vi "Initalize SR830(SubVI).vi"(0 "队列输入":refnum<queue>, 9 "字符串":string) -> ()   [LabVIEW 2019, in "SubVI.lvlib"]
uses:
  SubVI.lvlib
  lib/Keithley 622x/Configure/6221 Wave/Typedefs/KE6221 -- Wave Sine Wave Params.ctl
  lib/Keithley 622x/Configure/6221 Wave/Low Level/Typedefs/KE6221 -- Wave Frequency.ctl
  lib/Keithley 622x/Configure/6221 Wave/Low Level/Typedefs/KE6221 -- Wave Amplitude.ctl
  lib/Keithley 622x/Configure/Source/Typedefs/KE622x -- Current Level.ctl
  lib/Keithley 622x/Configure/6221 Wave/Low Level/Typedefs/KE6221 -- Wave Ranging Mode.ctl
  lib/Keithley 622x/Configure/Source/Typedefs/KE622x -- Current Ranges.ctl
  lib/Keithley 622x/Configure/6221 Wave/Low Level/Typedefs/KE6221 -- Wave Playback Mode.ctl
  lib/Keithley 622x/Configure/6221 Wave/Low Level/Typedefs/KE6221 -- Wave Playback Time.ctl
  lib/Keithley 622x/Configure/6221 Wave/Low Level/Typedefs/KE6221 -- Wave Playback Num Cycles.ctl
  lib/Keithley 622x/Configure/6221 Wave/Low Level/Typedefs/KE6221 -- Wave Phase Marker.ctl
  lib/Keithley 622x/Configure/Trigger/Low Level/Typedefs/KE622x -- Trig Link Line.ctl
  error.ctl
  lib/QDInstrument.dll
  lib/Keithley 622x/Configure/6221 Wave/Low Level/Typedefs/KE6221 -- Wave Type.ctl
  lib/Keithley 622x/Keithley 622x.lvlib
panel:
  out "x/y":dbl
  in  "6221(SR830做源可忽略）":T12={"Sine Wave Params In"={"Frequency (Hz)"=1000.0, "Amplitude (A)"=0.001, "Offset (A)"=0.0, "Ranging Mode"=enum."Best", "Fixed Range"=enum."2mA", "Playback Mode"=enum."Time", "Time (s)"=999999.999, "Num Cycles"=1.0, "Phase\nMarker?"=FALSE, "Phase Marker (deg)"=180.0, "Trig Link Line"=enum."1"}, "RMS Amplitude (A)"=0.001, "6221 resource"=""} {"RMS Amplitude (A)" min=2e-12 max=0.105 format="%.3p"; "Sine Wave Params In"."Offset (A)" min=-0.105 max=0.105 format="%.4p"; "Sine Wave Params In"."Num Cycles" min=0.001 max=99999999900.0 format="%.3p"; "Sine Wave Params In"."Time (s)" min=1e-07 max=999999.999 format="%.3p"; "Sine Wave Params In"."Phase Marker (deg)" min=0.0 max=360.0 format="%.3f"; "Sine Wave Params In"."Amplitude (A)" min=2e-12 max=0.105 format="%.3p"; "Sine Wave Params In"."Frequency (Hz)" min=0.001 max=100000.0 format="%.3p"}
  in  "仪器设置":T13={"ID Query"=FALSE, "Reset"=FALSE, "VISA 1"="", "VISA 2"="", "VISA 3"="", "VISA 4"="", "Sensitivity 2"=-1, "Sensitivity 1"=-1, "量程"=enum."量程每次测量会判定", "SR830源配合的阻抗（6221做源可忽略）"=0.0, "SR830 2"=FALSE, "SR830 3"=FALSE, "SR830 4"=FALSE, "Sensitivity 3"=-1, "Sensitivity 4"=-1, "source"=0, "SR830 1"=FALSE} {"source" items=["SR830 1", "SR830 2", "SR830 3", "SR830 4"]; "Sensitivity 4" items=["Auto Gain"=-1, "2 nV/fA"=0, "5 nV/fA"=1, "10 nV/fA"=2, "20 nV/fA"=3, "50 nV/fA"=4, "100 nV/fA"=5, "200 nV/fA"=6, "500 nV/fA"=7, "1 uV/pA"=8, "2 uV/pA"=9, "5 uV/pA"=10, "10 uV/pA"=11, "20 uV/pA"=12, "50 uV/pA"=13, "100 uV/pA"=14, "200 uV/pA"=15, "500 uV/pA"=16, "1 mV/nA"=17, "2 mV/nA"=18, "5 mV/nA"=19, "10 mV/nA"=20, "20 mV/nA"=21, "50 mV/nA"=22, "100 mV/nA"=23, "200 mV/nA"=24, "500 mV/mA"=25, "1 V/uA"=26]; "Sensitivity 3" items=["Auto Gain"=-1, "2 nV/fA"=0, "5 nV/fA"=1, "10 nV/fA"=2, "20 nV/fA"=3, "50 nV/fA"=4, "100 nV/fA"=5, "200 nV/fA"=6, "500 nV/fA"=7, "1 uV/pA"=8, "2 uV/pA"=9, "5 uV/pA"=10, "10 uV/pA"=11, "20 uV/pA"=12, "50 uV/pA"=13, "100 uV/pA"=14, "200 uV/pA"=15, "500 uV/pA"=16, "1 mV/nA"=17, "2 mV/nA"=18, "5 mV/nA"=19, "10 mV/nA"=20, "20 mV/nA"=21, "50 mV/nA"=22, "100 mV/nA"=23, "200 mV/nA"=24, "500 mV/mA"=25, "1 V/uA"=26]; "Sensitivity 1" items=["Auto Gain"=-1, "2 nV/fA"=0, "5 nV/fA"=1, "10 nV/fA"=2, "20 nV/fA"=3, "50 nV/fA"=4, "100 nV/fA"=5, "200 nV/fA"=6, "500 nV/fA"=7, "1 uV/pA"=8, "2 uV/pA"=9, "5 uV/pA"=10, "10 uV/pA"=11, "20 uV/pA"=12, "50 uV/pA"=13, "100 uV/pA"=14, "200 uV/pA"=15, "500 uV/pA"=16, "1 mV/nA"=17, "2 mV/nA"=18, "5 mV/nA"=19, "10 mV/nA"=20, "20 mV/nA"=21, "50 mV/nA"=22, "100 mV/nA"=23, "200 mV/nA"=24, "500 mV/mA"=25, "1 V/uA"=26]; "Sensitivity 2" items=["Auto Gain"=-1, "2 nV/fA"=0, "5 nV/fA"=1, "10 nV/fA"=2, "20 nV/fA"=3, "50 nV/fA"=4, "100 nV/fA"=5, "200 nV/fA"=6, "500 nV/fA"=7, "1 uV/pA"=8, "2 uV/pA"=9, "5 uV/pA"=10, "10 uV/pA"=11, "20 uV/pA"=12, "50 uV/pA"=13, "100 uV/pA"=14, "200 uV/pA"=15, "500 uV/pA"=16, "1 mV/nA"=17, "2 mV/nA"=18, "5 mV/nA"=19, "10 mV/nA"=20, "20 mV/nA"=21, "50 mV/nA"=22, "100 mV/nA"=23, "200 mV/nA"=24, "500 mV/mA"=25, "1 V/uA"=26]}
  out "错误输出":errorcluster
  in  "滤波设置 4":T14={"Time Constant "=8, "Low Pass Filter Slope "=1, "Enable Sync Filter "=TRUE} {"Low Pass Filter Slope" items=["6 dB/oct", "12 dB/oct", "18 db/oct", "24 dB/oct"]; "Time Constant" items=["10 us", "30 us", "100 us", "300 us", "1 ms", "3 ms", "10 ms", "30 ms", "100 ms", "300 ms", "1 s", "3 s", "10 s", "30 s", "100 s", "300 s", "1 ks", "3 ks", "10 ks", "30 ks"]}
  in  "滤波设置 3":T14={"Time Constant "=8, "Low Pass Filter Slope "=1, "Enable Sync Filter "=TRUE} {"Low Pass Filter Slope" items=["6 dB/oct", "12 dB/oct", "18 db/oct", "24 dB/oct"]; "Time Constant" items=["10 us", "30 us", "100 us", "300 us", "1 ms", "3 ms", "10 ms", "30 ms", "100 ms", "300 ms", "1 s", "3 s", "10 s", "30 s", "100 s", "300 s", "1 ks", "3 ks", "10 ks", "30 ks"]}
  in  "滤波设置 2":T14={"Time Constant "=8, "Low Pass Filter Slope "=1, "Enable Sync Filter "=TRUE} {"Low Pass Filter Slope" items=["6 dB/oct", "12 dB/oct", "18 db/oct", "24 dB/oct"]; "Time Constant" items=["10 us", "30 us", "100 us", "300 us", "1 ms", "3 ms", "10 ms", "30 ms", "100 ms", "300 ms", "1 s", "3 s", "10 s", "30 s", "100 s", "300 s", "1 ks", "3 ks", "10 ks", "30 ks"]}
  in  "参考信号 4":T15={"Reference Source"=1, "External Reference Trigger  "=0, "Detection Harmonic Number "=1.0, "Manual Phase (Degree)"=0.0, "Auto Phase "=FALSE, "Sine Output Amplitude (V)"=1.0, "Internal Reference Frequency (Hz)"=13.0} {"External Reference Trigger" items=["Sine Zero Crossing", "TTL Rising Edge", "TTL Falling Edge"]; "Reference Source" items=["External", "Internal"]}
  in  "参考信号 3":T15={"Reference Source"=1, "External Reference Trigger  "=0, "Detection Harmonic Number "=1.0, "Manual Phase (Degree)"=0.0, "Auto Phase "=FALSE, "Sine Output Amplitude (V)"=1.0, "Internal Reference Frequency (Hz)"=13.0} {"External Reference Trigger" items=["Sine Zero Crossing", "TTL Rising Edge", "TTL Falling Edge"]; "Reference Source" items=["External", "Internal"]}
  in  "参考信号 2":T15={"Reference Source"=1, "External Reference Trigger  "=0, "Detection Harmonic Number "=1.0, "Manual Phase (Degree)"=0.0, "Auto Phase "=FALSE, "Sine Output Amplitude (V)"=1.0, "Internal Reference Frequency (Hz)"=13.0} {"External Reference Trigger" items=["Sine Zero Crossing", "TTL Rising Edge", "TTL Falling Edge"]; "Reference Source" items=["External", "Internal"]}
  in  "输入信号 4":T16={"Input Notch Filter "=0, "Input Shield Grounding"=0, "Input Coupling "=0, "Input Connection  "=1} {"Input Connection" items=["Single-Ended Voltage", "Differential Voltage", "1 MOhm Current Gain", "100 MOhm Current Gain"]; "Input Coupling" items=["AC", "DC"]; "Input Shield Grounding" items=["Float", "Ground"]; "Input Notch Filter" items=["None", "Line Notch", "2x Line Notch", "Both Notch Filters"]}
  in  "输入信号 3":T16={"Input Notch Filter "=0, "Input Shield Grounding"=0, "Input Coupling "=0, "Input Connection  "=1} {"Input Connection" items=["Single-Ended Voltage", "Differential Voltage", "1 MOhm Current Gain", "100 MOhm Current Gain"]; "Input Coupling" items=["AC", "DC"]; "Input Shield Grounding" items=["Float", "Ground"]; "Input Notch Filter" items=["None", "Line Notch", "2x Line Notch", "Both Notch Filters"]}
  in  "输入信号 2":T16={"Input Notch Filter "=0, "Input Shield Grounding"=0, "Input Coupling "=0, "Input Connection  "=1} {"Input Connection" items=["Single-Ended Voltage", "Differential Voltage", "1 MOhm Current Gain", "100 MOhm Current Gain"]; "Input Coupling" items=["AC", "DC"]; "Input Shield Grounding" items=["Float", "Ground"]; "Input Notch Filter" items=["None", "Line Notch", "2x Line Notch", "Both Notch Filters"]}
  in  "滤波设置":T14={"Time Constant "=8, "Low Pass Filter Slope "=1, "Enable Sync Filter "=TRUE} {"Low Pass Filter Slope" items=["6 dB/oct", "12 dB/oct", "18 db/oct", "24 dB/oct"]; "Time Constant" items=["10 us", "30 us", "100 us", "300 us", "1 ms", "3 ms", "10 ms", "30 ms", "100 ms", "300 ms", "1 s", "3 s", "10 s", "30 s", "100 s", "300 s", "1 ks", "3 ks", "10 ks", "30 ks"]}
  in  "参考信号":T15={"Reference Source"=1, "External Reference Trigger  "=0, "Detection Harmonic Number "=1.0, "Manual Phase (Degree)"=0.0, "Auto Phase "=FALSE, "Sine Output Amplitude (V)"=1.0, "Internal Reference Frequency (Hz)"=13.0} {"External Reference Trigger" items=["Sine Zero Crossing", "TTL Rising Edge", "TTL Falling Edge"]; "Reference Source" items=["External", "Internal"]}
  in  "输入信号":T16={"Input Notch Filter "=0, "Input Shield Grounding"=0, "Input Coupling "=0, "Input Connection  "=1} {"Input Connection" items=["Single-Ended Voltage", "Differential Voltage", "1 MOhm Current Gain", "100 MOhm Current Gain"]; "Input Coupling" items=["AC", "DC"]; "Input Shield Grounding" items=["Float", "Ground"]; "Input Notch Filter" items=["None", "Line Notch", "2x Line Notch", "Both Notch Filters"]}
  # "(真是通道1，假是通道2)"
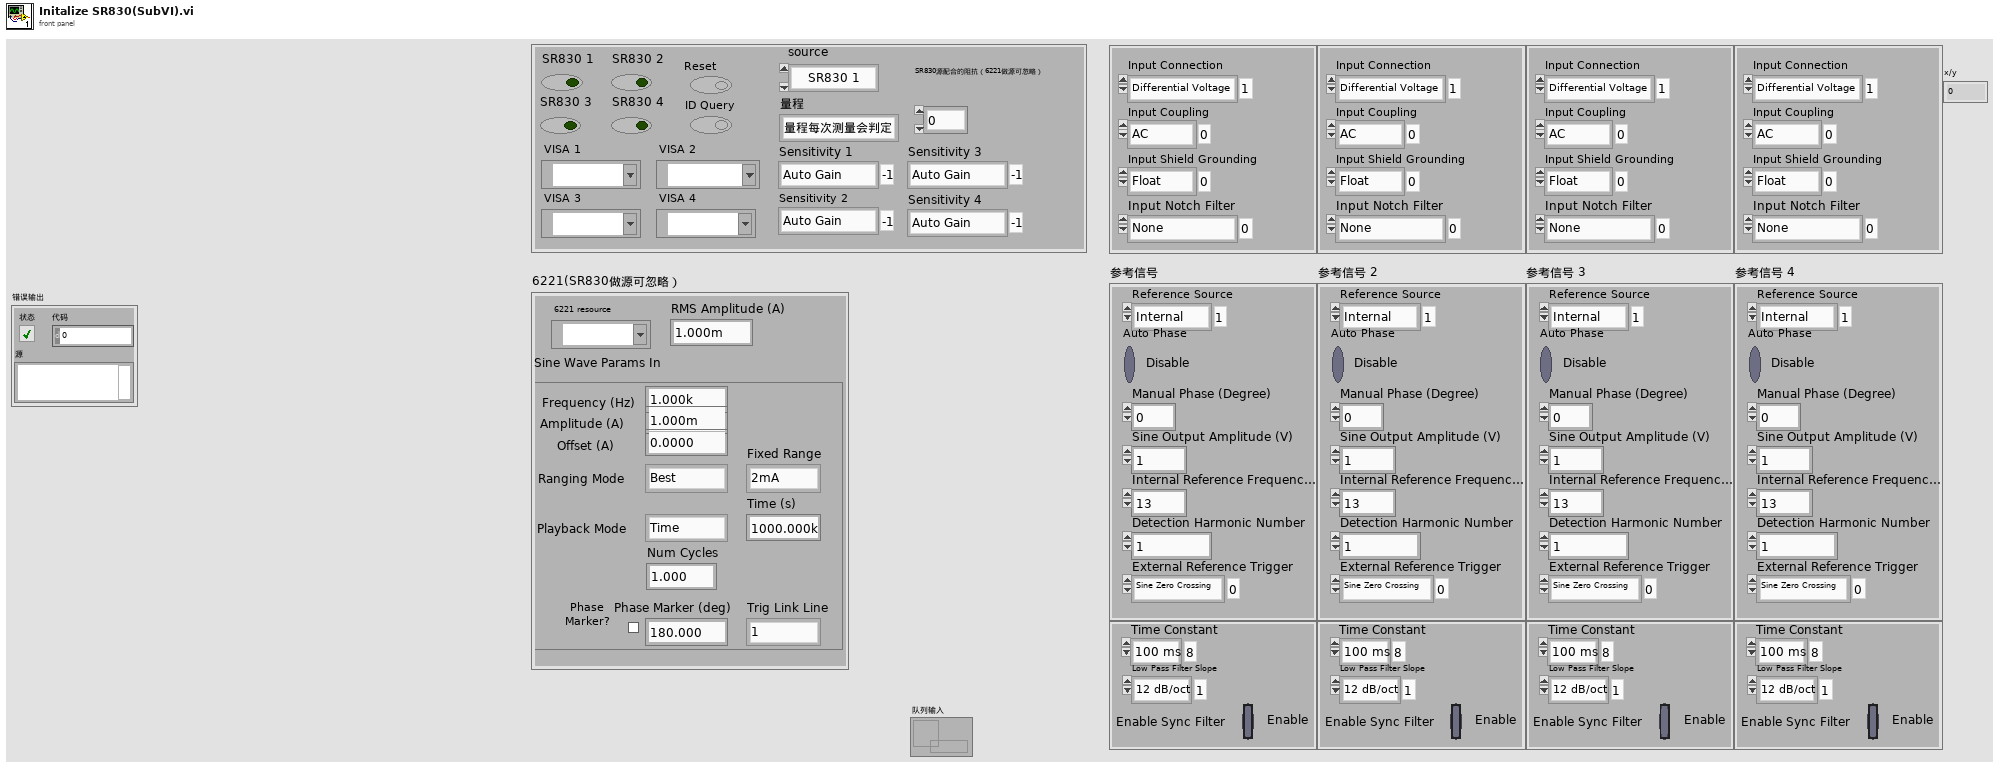
[diagram p1: front panel]
types:
  T1 = typedef "Keithley 622x.lvlib/KE6221 -- Wave Sine Wave Params.ctl" = cluster{"Frequency (Hz)":T2, "Amplitude (A)":T3, "Offset (A)":T4, "Ranging Mode":T5, "Fixed Range":T6, "Playback Mode":T7, "Time (s)":T8, "Num Cycles":T9, "Phase\nMarker?":bool, "Phase Marker (deg)":T10, "Trig Link Line":T11}
  T2 = typedef "Keithley 622x.lvlib/KE6221 -- Wave Frequency.ctl" = dbl
  T3 = typedef "Keithley 622x.lvlib/KE6221 -- Wave Amplitude.ctl" = dbl
  T4 = typedef "Keithley 622x.lvlib/KE622x -- Current Level.ctl" = dbl
  T5 = typedef "Keithley 622x.lvlib/KE6221 -- Wave Ranging Mode.ctl" = enum16{"Best", "Fixed"}
  T6 = typedef "Keithley 622x.lvlib/KE622x -- Current Ranges.ctl" = enum16{"2nA", "20nA", "200nA", "2uA", "20uA", "200uA", "2mA", "20mA", "100mA"}
  T7 = typedef "Keithley 622x.lvlib/KE6221 -- Wave Playback Mode.ctl" = enum16{"Time", "Num Cycles"}
  T8 = typedef "Keithley 622x.lvlib/KE6221 -- Wave Playback Time.ctl" = dbl
  T9 = typedef "Keithley 622x.lvlib/KE6221 -- Wave Playback Num Cycles.ctl" = dbl
  T10 = typedef "Keithley 622x.lvlib/KE6221 -- Wave Phase Marker.ctl" = dbl
  T11 = typedef "Keithley 622x.lvlib/KE622x -- Trig Link Line.ctl" = enum16{"1", "2", "3", "4", "5", "6"}
  T12 = cluster{"Sine Wave Params In":T1, "RMS Amplitude (A)":T3, "6221 resource":refnum<visa-resource-name>}
  T13 = cluster{"ID Query":bool, "Reset":bool, "VISA 1":refnum<visa-resource-name>, "VISA 2":refnum<visa-resource-name>, "VISA 3":refnum<visa-resource-name>, "VISA 4":refnum<visa-resource-name>, "Sensitivity 2":i16, "Sensitivity 1":i16, "量程":enum16{"量程每次测量会判定", "量程不变为设定值"}, "SR830源配合的阻抗（6221做源可忽略）":dbl, "SR830 2":bool, "SR830 3":bool, "SR830 4":bool, "Sensitivity 3":i16, "Sensitivity 4":i16, "source":u16, "SR830 1":bool}
  T14 = cluster{"Time Constant ":u16, "Low Pass Filter Slope ":u16, "Enable Sync Filter ":bool}
  T15 = cluster{"Reference Source":u16, "External Reference Trigger  ":u16, "Detection Harmonic Number ":dbl, "Manual Phase (Degree)":dbl, "Auto Phase ":bool, "Sine Output Amplitude (V)":dbl, "Internal Reference Frequency (Hz)":dbl}
  T16 = cluster{"Input Notch Filter ":u16, "Input Shield Grounding":u16, "Input Coupling ":u16, "Input Connection  ":u16}
  T17 = enum16{"open", "replace", "create", "open or create", "replace or create", "replace or create with confirmation"}
  T18 = typedef "Keithley 622x.lvlib/KE6221 -- Wave Type.ctl" = enum16{"Sinusoid", "Square", "Ramp", "Arbitrary 0", "Arbitrary 1", "Arbitrary 2", "Arbitrary 3", "Arbitrary 4"}
  T19 = typedef "Keithley 622x.lvlib/KE622x -- On Off Control.ctl" = enum16{"Off", "On"}
  T20 = typedef "error.ctl" = cluster{"initialize":string, "6221":cluster{"6221 Resource":refnum<visa-resource-name>, "Delta status":bool}, "7001":cluster{"Ch":bool}, "SR830+6221":cluster{"source":u16, "阻抗":dbl, "量程入 4":i32, "量程入 3":i32, "量程入 2":i32, "量程入 1":i32, "电流":dbl, "SR830 2":bool, "SR830 3":bool, "SR830 4":bool, "SR830 1":bool, "VISA 1":refnum<visa-resource-name>, "VISA 2":refnum<visa-resource-name>, "VISA 3":refnum<visa-resource-name>, "VISA 4":refnum<visa-resource-name>, "量程":enum16{"量程每次测量会判定", "量程不变为设定值"}}, "2400":cluster{"2400":bool, "VISA":refnum<visa-resource-name>}, "ch":cluster{"ch str":string, "ch1":bool, "ch2":bool, "布尔":bool}, "quantum design":refnum<k24>, "error":bool, "数据文件路径":path, "簇":cluster{"log路径":path, "log interval":dbl}}
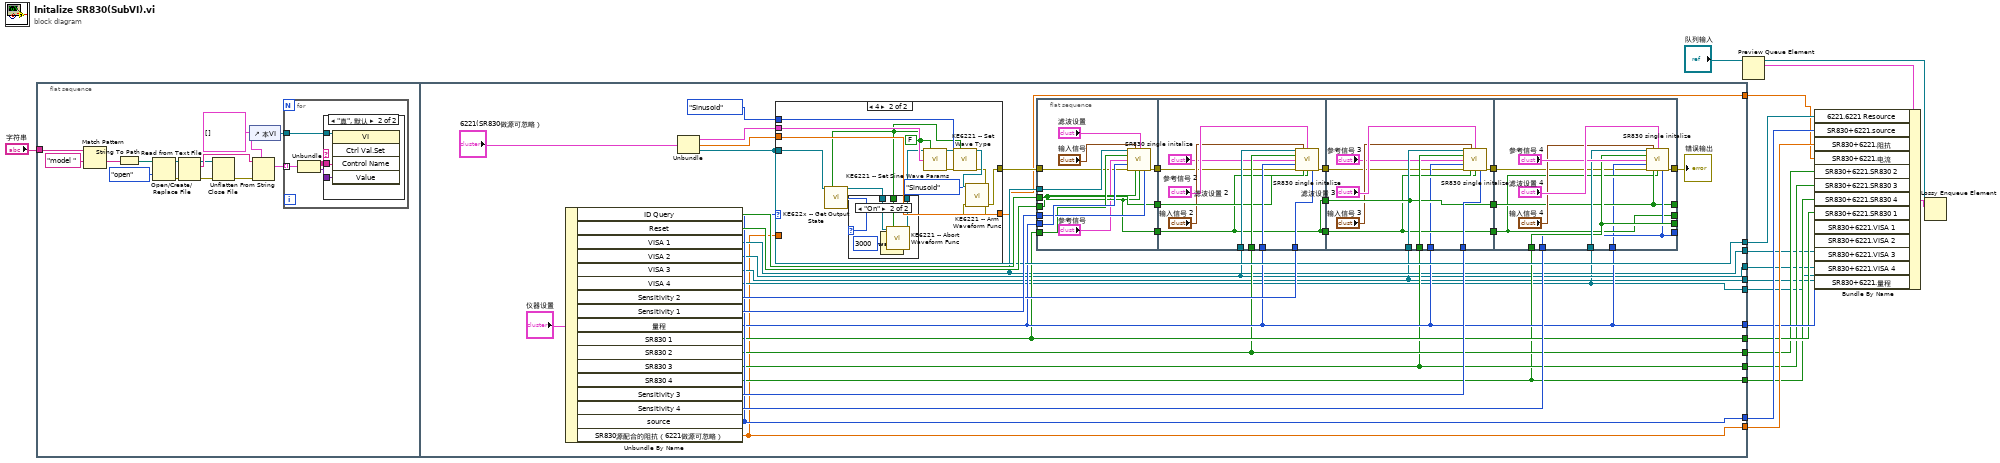
[diagram p0: block diagram]
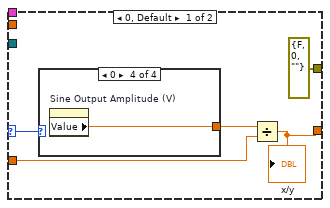
[diagram p3: hidden frame]
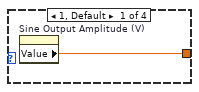
[diagram p4: hidden frame]
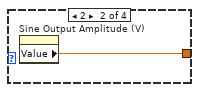
[diagram p5: hidden frame]
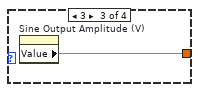
[diagram p6: hidden frame]
diagram:
  n1 = flat-sequence {
    tunnel: "字符串" -> [w32]
    tunnel: [w56] -> w13
    tunnel: [w53] -> w14
    tunnel: [w41] -> w12
    tunnel: [w51] -> w10
    tunnel: [w50] -> w9
    tunnel: [w49] -> w8
    tunnel: [w48] -> w7
    tunnel: [w47] -> w6
    tunnel: [w46] -> w5
    tunnel: [w45] -> w4
    tunnel: [w44] -> w3
    tunnel: [w43] -> w2
    tunnel: [w40] -> w1
    frame #0 {
      n2 = Match Pattern(string=w32, regular expression="model " ("正则表达式")) -> (after substring=w31:string)  [unwired: 1 in, 3 out]
      n3 = String To Path(string=w31) -> (path=w30:path)
      n4 = Open/Create/Replace File(file path (use dialog)=w30, operation (0:open)=T17."open" ("操作(0:open)")) -> (refnum out=w27:refnum<file>, error out=w25:errorcluster)  [unwired: 4 in, 1 out]
      n5 = Read from Text File(file (use dialog)=w27, error in=w25) -> (refnum out=w26:refnum<file>, text=w28:string, error out=w24:errorcluster)  [unwired: 2 in, 1 out]
      n6 = Close File(refnum=w26, error in=w24) -> (error out=w23:errorcluster)  [unwired: 1 out]
      n7 = control-ref of="本VI"() -> (w19:refnum<vi>)
      n8 = Unflatten From String(type=cluster{"Name":string, "Variant Data":variant}[] [] ("控件值:获取全部"), binary string=w28, error in (no error)=w23) -> (value=w20:cluster{"Name":string, "Variant Data":variant}[])  [unwired: 2 in, 2 out]
      n9 = for {
        tunnel: w20 -> [w36] mode=indexing
        tunnel: w19 -> [w35]
        n10 = Unbundle(w36) -> ("Name"=w33:string, "Variant Data"=w34:variant)
        n11 = case shown="\"真\", 默认" w33 {
          tunnel: w35 -> [_ w39]
          tunnel: w33 -> [_ w38]
          tunnel: w34 -> [_ w37]
          frame "cancel", "load", "model", "ok" {
          }
          frame "真", Default {
            n12 = invoke class="VI" method="Ctrl Val.Set"(reference=w39, "Control Name"=w38, "Value"=w37) -> ()  [unwired: 2 in, 5 out]
          }
        }
      }
    }
    frame #1 {
      n13 = Unbundle By Name("仪器设置") -> ("ID Query"=w73:bool, "Reset"=w72:bool, "VISA 1"=w46:refnum<visa-resource-name>, "VISA 2"=w45:refnum<visa-resource-name>, "VISA 3"=w44:refnum<visa-resource-name>, "VISA 4"=w43:refnum<visa-resource-name>, "Sensitivity 2"=w69:i16, "Sensitivity 1"=w74:i16, "量程"=w51:enum16{"量程每次测量会判定", "量程不变为设定值"}, "SR830 1"=w50:bool, "SR830 2"=w49:bool, "SR830 3"=w48:bool, "SR830 4"=w47:bool, "Sensitivity 3"=w71:i16, "Sensitivity 4"=w70:i16, "source"=w56:u16, "SR830源配合的阻抗（6221做源可忽略）"=w41:dbl)
      n14 = Unbundle("6221(SR830做源可忽略）") -> ("Sine Wave Params In"=w54:T1, "RMS Amplitude (A)"=w42:T3, "6221 resource"=w53:refnum<visa-resource-name>)
      n15 = case shown="4" w56 {
        selector: w56 -> [w76 _]
        tunnel: KE6221_--_Wave_Type."Sinusoid" ("Wave Type") -> [_ w97]
        tunnel: [errorcluster {"status"=FALSE, "code"=0, "source"=""} ("error out") w90] -> w57
        tunnel: w54 -> [_ w94]
        tunnel: w53 -> [_ w89]
        tunnel: w42 -> [_ w93]
        tunnel: w41 -> [w77 _]
        tunnel: [w75 w93] -> w40
        frame 0, Default {
          n16 = case shown="0" w76 {
            tunnel: [w80 w81 w82 w83] -> w78
            frame 1, Default {
              n17 = property on="Sine Output Amplitude (V)" class="DigNum (严格)"() -> ("Value"=w80:dbl)  [unwired: 2 in, 2 out]
            }
            frame 2 {
              n18 = property on="Sine Output Amplitude (V)" class="DigNum (严格)"() -> ("Value"=w81:dbl)  [unwired: 2 in, 2 out]
            }
            frame 3 {
              n19 = property on="Sine Output Amplitude (V)" class="DigNum (严格)"() -> ("Value"=w82:dbl)  [unwired: 2 in, 2 out]
            }
            frame 0 {
              n20 = property on="Sine Output Amplitude (V)" class="DigNum (严格)"() -> ("Value"=w83:dbl)  [unwired: 2 in, 2 out]
            }
          }
          n21 = Divide(x=w78, y=w77) -> (x/y=w75:dbl)
          "x/y" <- w75
        }
        frame 4 {
          w86 = FALSE ("Check For SCPI Errors? (T)")
          n22 = call "KE622x -- Get Output State.vi"("Resource In"=w89, "Check For SCPI Errors? (T)"=w86) -> ("Resource Out (dupl)"=w87:refnum<visa-resource-name>, "Output State"=w88:T19)  [unwired: 11 in, 1 out]
          n23 = case shown="\"On\"" w88 {
            tunnel: w87 -> [w98 w102]
            tunnel: w86 -> [_ w101]
            tunnel: [w98 w100] -> w85
            frame "Off", Default {
            }
            frame "On" {
              n24 = Wait (ms)(milliseconds to wait=u32 3000 ("等待时间（毫秒）")) -> ()  [unwired: 1 out]
              n25 = call "KE6221 -- Abort Waveform Func.vi"("Resource In"=w102, "Check For SCPI Errors? (T)"=w101) -> ("Resource Out (dupl)"=w100:refnum<visa-resource-name>)  [unwired: 12 in, 1 out]
            }
          }
          n26 = call "KE6221 -- Set Sine Wave Params.vi"("Resource In"=w85, "Check For SCPI Errors? (T)"=w86, "Sine Wave Params In"=w94) -> ("Resource Out (dupl)"=w96:refnum<visa-resource-name>, "error out"=w95:errorcluster)  [unwired: 10 in, 1 out]
          n27 = call "KE6221 -- Set Wave Type.vi"("Resource In"=w96, "Check For SCPI Errors? (T)"=w86, "Wave Type"=w97, "error in (no error)"=w95) -> ("Resource Out (dupl)"=w92:refnum<visa-resource-name>, "error out"=w91:errorcluster)  [unwired: 10 in]
          n28 = call "KE6221 -- Arm Waveform Func.vi"("Resource In"=w92, "Wave Type"=KE6221_--_Wave_Type."Sinusoid", "error in (no error)"=w91) -> ("error out"=w90:errorcluster)  [unwired: 11 in, 1 out]
        }
      }
      n29 = flat-sequence {
        tunnel: w46 -> [w113]
        tunnel: w51 -> [w112]
        tunnel: w74 -> [w111]
        tunnel: w73 -> [w109]
        tunnel: w72 -> [w108]
        tunnel: w50 -> [w110]
        tunnel: [w109] -> w68
        tunnel: [w108] -> w67
        tunnel: [w104] -> w62
        tunnel: w57 -> [w103]
        tunnel: w45 -> [w124]
        tunnel: w49 -> [w123]
        tunnel: w69 -> [w122]
        tunnel: w51 -> [w121]
        tunnel: w68 -> [w120]
        tunnel: w67 -> [w119]
        tunnel: [w119] -> w66
        tunnel: [w119] -> w65
        tunnel: w62 -> [w115]
        tunnel: [w114] -> w61
        tunnel: w44 -> [w135]
        tunnel: w48 -> [w134]
        tunnel: w71 -> [w133]
        tunnel: w66 -> [w132]
        tunnel: w65 -> [w131]
        tunnel: [w132] -> w64
        tunnel: [w131] -> w63
        tunnel: w51 -> [w130]
        tunnel: w61 -> [w126]
        tunnel: [w125] -> w60
        tunnel: [w142] -> _
        tunnel: [w139] -> _
        tunnel: [w140] -> _
        tunnel: [w141] -> _
        tunnel: w43 -> [w143]
        tunnel: w47 -> [w142]
        tunnel: w70 -> [w141]
        tunnel: w64 -> [w140]
        tunnel: w63 -> [w139]
        tunnel: w51 -> [w138]
        tunnel: w60 -> [w137]
        tunnel: [w136] -> w59
        frame #0 {
          n30 = call "SR830 single initalize.vi"("VISA引用句柄输入"=w113, "输入信号"="输入信号", "滤波设置"="滤波设置", "open"=w110, "参考信号"="参考信号", "量程"=w112, "error in (no error)"=w103, "ID Query (True)"=w109, "Reset (True)"=w108, "Sensitivity (-1: Auto gain)"=w111) -> ("错误输出"=w104:cluster{"status":bool, "code":i32, string})  [unwired: 5 in]
        }
        frame #1 {
          n31 = call "SR830 single initalize.vi"("VISA引用句柄输入"=w124, "输入信号"="输入信号 2", "滤波设置"="滤波设置 2", "open"=w123, "参考信号"="参考信号 2", "量程"=w121, "error in (no error)"=w115, "ID Query (True)"=w120, "Reset (True)"=w119, "Sensitivity (-1: Auto gain)"=w122) -> ("错误输出"=w114:cluster{"status":bool, "code":i32, string})  [unwired: 5 in]
        }
        frame #2 {
          n32 = call "SR830 single initalize.vi"("VISA引用句柄输入"=w135, "输入信号"="输入信号 3", "滤波设置"="滤波设置 3", "open"=w134, "参考信号"="参考信号 3", "量程"=w130, "error in (no error)"=w126, "ID Query (True)"=w132, "Reset (True)"=w131, "Sensitivity (-1: Auto gain)"=w133) -> ("错误输出"=w125:cluster{"status":bool, "code":i32, string})  [unwired: 5 in]
        }
        frame #3 {
          n33 = call "SR830 single initalize.vi"("VISA引用句柄输入"=w143, "输入信号"="输入信号 4", "滤波设置"="滤波设置 4", "open"=w142, "参考信号"="参考信号 4", "量程"=w138, "error in (no error)"=w137, "ID Query (True)"=w140, "Reset (True)"=w139, "Sensitivity (-1: Auto gain)"=w141) -> ("错误输出"=w136:cluster{"status":bool, "code":i32, string})  [unwired: 5 in]
        }
      }
      "错误输出" <- w59
    }
  }
  n34 = Preview Queue Element(queue="队列输入") -> (queue out=w16:refnum<queue>, element=w17:T20)  [unwired: 2 in, 2 out]
  n35 = Bundle By Name(cluster=w17, "6221.6221 Resource"=w14, "SR830+6221.source"=w13, "SR830+6221.阻抗"=w12, "SR830+6221.电流"=w1, "SR830+6221.SR830 2"=w8, "SR830+6221.SR830 3"=w7, "SR830+6221.SR830 4"=w6, "SR830+6221.SR830 1"=w9, "SR830+6221.VISA 1"=w5, "SR830+6221.VISA 2"=w4, "SR830+6221.VISA 3"=w3, "SR830+6221.VISA 4"=w2, "SR830+6221.量程"=w10) -> (w15:T20)
  n36 = Lossy Enqueue Element(queue=w16, element=w15) -> ()  [unwired: 1 in, 4 out]
